vi "globalsd.vi"() -> ()   [LabVIEW 2017]
panel:
  in  "Dead":bool
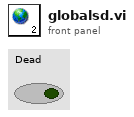
[diagram p1: front panel]
diagram:
